vi "test_read_digital_worker.vi"() -> ()   [LabVIEW 2017]
uses:
  hardware/hardware_type.ctl
  support/Message Queue/Enqueue Message (Single).vi
  <vilib>/Utility/error.llb/Error Cluster From Error Code.vi
  <vilib>/ErrorRing/Error Ring.xnode
  measurement_data/MeasurementDatalvclass.lvclass
  support/Message Queue/Message Queue.lvlib
  support/User Event - Stop/User Event - Stop.lvlib
  logger/logger.lvlib
  hardware/Hardware.lvclass
panel:
  in  "hardware type":T1
  out "time_stamp":timestamp
  out "raw_data":u16[][](array[numeric])
  in  "stop":bool
  in  "Play Button":bool
  out "status":string
  in  "Exit":bool
  # "row is channel and col is sample / channel"
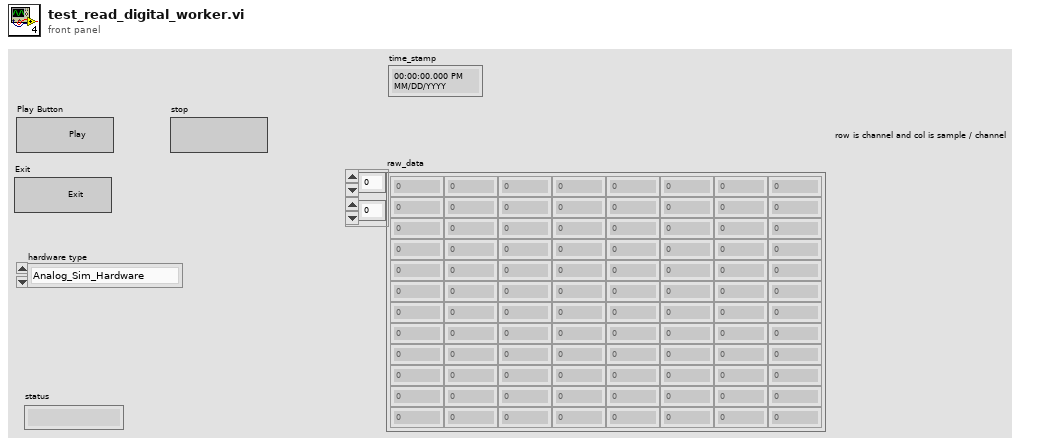
[diagram p1: front panel]
types:
  T1 = typedef "Hardware.lvclass/hardware_type.ctl" = enum16{"Analog_Sim_Hardware", "Digital_Sim_Hardware", "AI_Ni_Hardware", "AO_Ni_Hardware", "DI_Ni_Hardware", "DO_Ni_Hardware"}
  T2 = typedef "Message Queue.lvlib/All Message Queues.ctl" = cluster{"MHL":refnum<queue>, "TCPServerLoop":refnum<queue>, "RequestProcessorLoop":refnum<queue>, "AnalogReadWorkerLoop":refnum<queue>, "AnalogWriteWorkerLoop":refnum<queue>, "DigitalReadWorkerLoop":refnum<queue>, "DigitalWriteWorkerLoop":refnum<queue>}
  T3 = typedef "Notifiers.ctl" = cluster{"TCPServerExit":refnum<notifier>, "RequestProcesscorExit":refnum<notifier>, "AnalogReadWorkerrExit":refnum<notifier>, "AnalogWriteWorkerrExit":refnum<notifier>, "DigitalReadWorkerrExit":refnum<notifier>, "DigitalWriteWorkerrExit":refnum<notifier>}
  T4 = typedef "data_Notifiers.ctl" = cluster{"AnalogReadResult":refnum<notifier>}
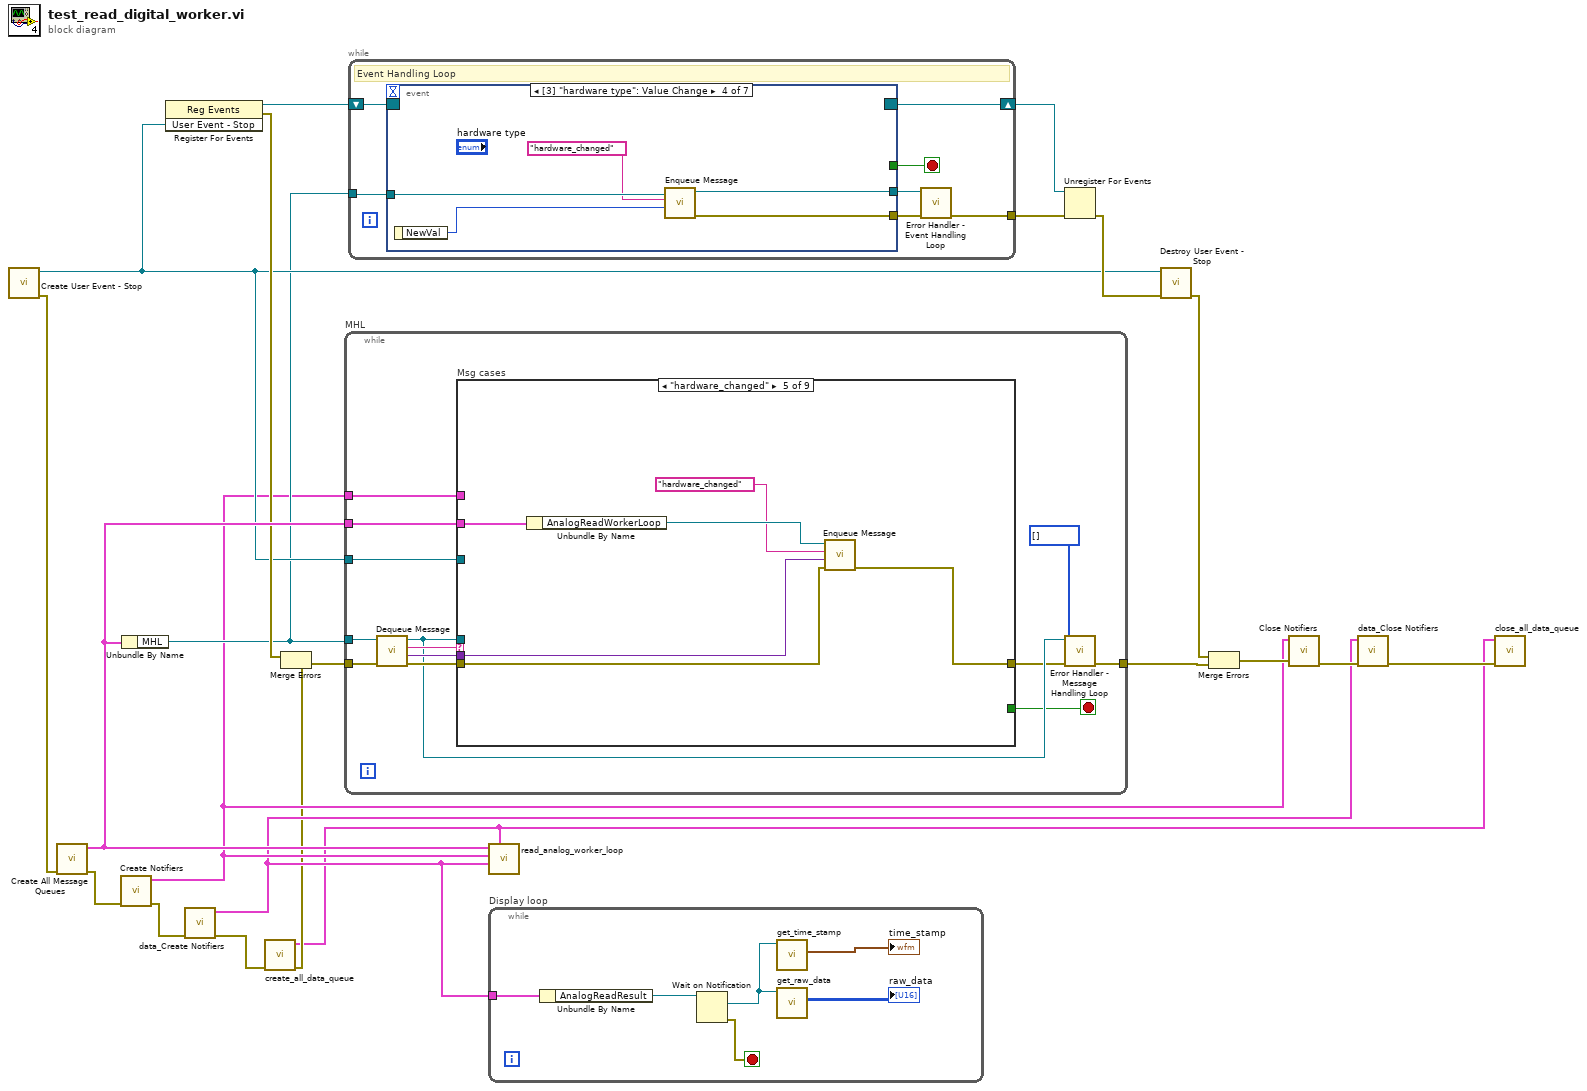
[diagram p0: block diagram]
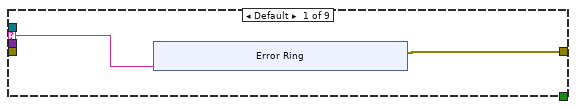
[diagram p2: hidden frame]
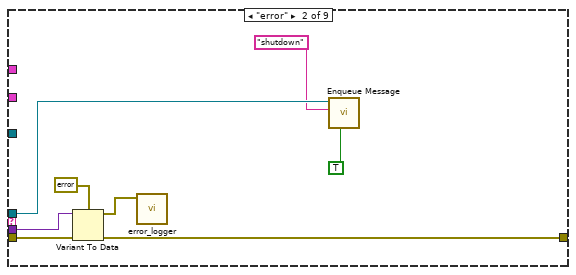
[diagram p3: hidden frame]
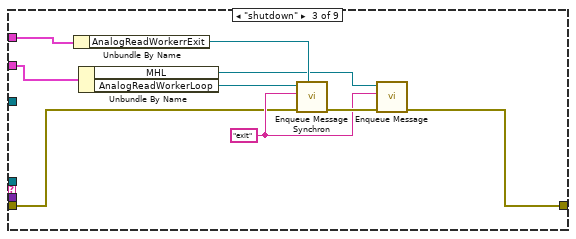
[diagram p4: hidden frame]
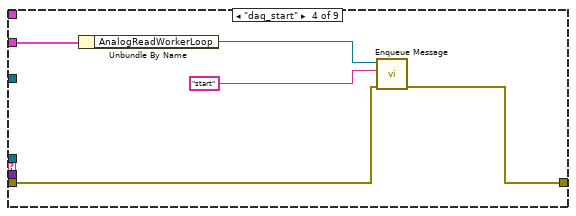
[diagram p5: hidden frame]
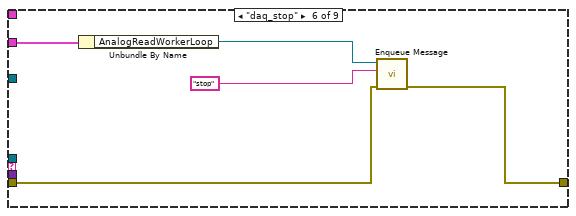
[diagram p6: hidden frame]
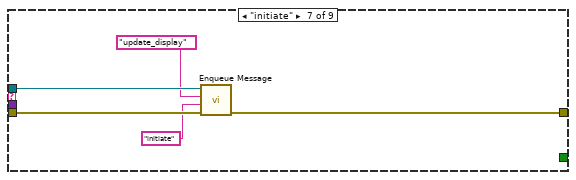
[diagram p7: hidden frame]
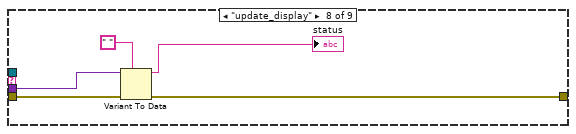
[diagram p8: hidden frame]
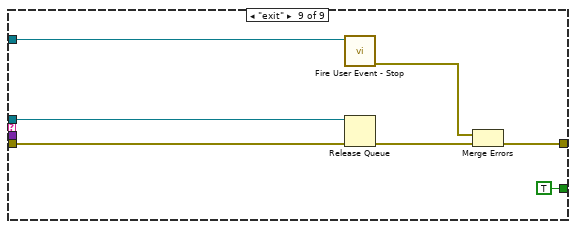
[diagram p9: hidden frame]
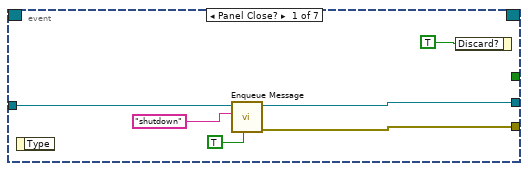
[diagram p10: hidden frame]
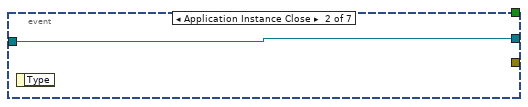
[diagram p11: hidden frame]
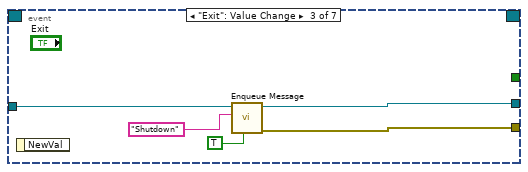
[diagram p12: hidden frame]
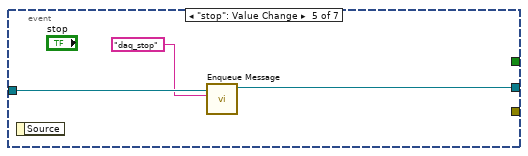
[diagram p13: hidden frame]
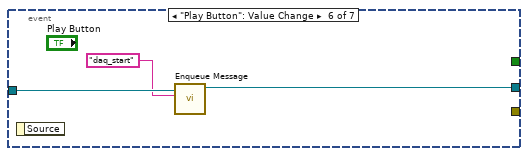
[diagram p14: hidden frame]
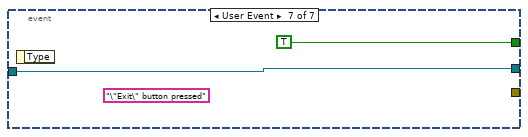
[diagram p15: hidden frame]
diagram:
  n1 = call "Create User Event - Stop.vi"() -> ("error out"=w17:errorcluster, "User Event - Stop"=w12:refnum<user-event>)  [unwired: 10 in]
  n2 = call "Create All Message Queues.vi"("error in (no error)"=w17) -> ("error out"=w16:errorcluster, "Message Queues out"=w18:T2)  [unwired: 9 in]
  n3 = call "Create Notifiers.vi"("error in"=w16) -> ("error out"=w15:errorcluster, "Notifiers"=w6:T3)  [unwired: 9 in]
  n4 = Unbundle By Name(w18) -> ("MHL"=w11:refnum<queue>)
  n5 = register-events(w12) -> (reference out=w21:refnum<event-registration>, error out=w13:errorcluster)  [unwired: 2 in]
  n6 = call "data_Create Notifiers.vi"("error in"=w15) -> ("error out"=w4:errorcluster, "output cluster"=w5:T4)  [unwired: 9 in]
  n7 = call "create_all_data_queue.vi"("error in (no error)"=w4) -> ("error out"=w3:errorcluster, "data_queue"=w1:cluster{"AnalogReadData":refnum<queue>})  [unwired: 9 in]
  n8 = Merge Errors(w13, w3) -> (w14:errorcluster)
  n9 = while "MHL" {
    tunnel: w14 -> [w32]
    tunnel: w11 -> [w31]
    tunnel: w18 -> [w30]
    tunnel: w12 -> [w29]
    tunnel: w6 -> [w25]
    tunnel: [w24] -> w8
    stop <- w26 stop-if-true
    n10 = call "Dequeue Message.vi"("error in (no error)"=w32, "Message Queue"=w31) -> ("error out"=w33:errorcluster, "Message Data"=w34:variant, "Message"=w35:string, "dup Message Queue"=w28:refnum<queue>)  [unwired: 6 in]
    n11 = case "Msg cases" shown="\"hardware_changed\"" w35 {
      selector: w35 -> [w37 _ _ _ _ _ _ _ _]
      tunnel: w28 -> [_ w52 _ _ _ _ w79 _ w92]
      tunnel: w34 -> [_ w47 _ _ w67 _ _ w85 _]
      tunnel: w33 -> [_ w46 w53 w62 w68 w73 w82 w87 w93]
      tunnel: w30 -> [_ _ w59 w66 w72 w77 _ _ _]
      tunnel: w29 -> [_ _ _ _ _ _ _ _ w91]
      tunnel: [w36 w45 w54 w63 w69 w74 w81 w86 w88] -> w27
      tunnel: [_ _ _ _ _ _ _ _ TRUE] -> w26
      tunnel: w25 -> [_ _ w61 _ _ _ _ _ _]
      frame Default {
        n12 = xnode "Error Ring"("parameter 0"=w37) -> ("error out"=w36:errorcluster)
      }
      frame "error" {
        n13 = Variant To Data(error in=w46, type=errorcluster {"status"=FALSE, "code"=0, "source"=""} ("error constant"), Variant=w47) -> (data=w48:errorcluster, error out=w45:errorcluster)
        n14 = call "error_logger.vi"("error in (no error)"=w48) -> ()  [unwired: 11 in]
        n15 = call-poly "Enqueue Message.vi"("Priority Message? (F)"=TRUE, "Message"="shutdown", "Message Queue"=w52) -> ()  [unwired: 7 in, 2 out]
      }
      frame "shutdown" {
        w55 = "exit"
        n16 = Unbundle By Name(w61) -> ("AnalogReadWorkerrExit"=w60:refnum<notifier>)
        n17 = Unbundle By Name(w59) -> ("MHL"=w57:refnum<queue>, "AnalogReadWorkerLoop"=w58:refnum<queue>)
        n18 = call "Enqueue Message Synchron.vi"("Notifier"=w60, "error in (no error)"=w53, "Message"=w55, "Message Queue"=w58) -> ("error out"=w56:errorcluster)  [unwired: 6 in, 1 out]
        n19 = call-poly "Enqueue Message.vi"("error in (no error)"=w56, "Message"=w55, "Message Queue"=w57) -> ("error out"=w54:errorcluster)  [unwired: 7 in, 1 out]
      }
      frame "daq_start" {
        n20 = Unbundle By Name(w66) -> ("AnalogReadWorkerLoop"=w65:refnum<queue>)
        n21 = call-poly "Enqueue Message.vi"("error in (no error)"=w62, "Message"="start", "Message Queue"=w65) -> ("error out"=w63:errorcluster)  [unwired: 7 in, 1 out]
      }
      frame "hardware_changed" {
        n22 = Unbundle By Name(w72) -> ("AnalogReadWorkerLoop"=w71:refnum<queue>)
        n23 = call-poly "Enqueue Message.vi"("error in (no error)"=w68, "Message Data"=w67, "Message"="hardware_changed", "Message Queue"=w71) -> ("error out"=w69:errorcluster)  [unwired: 6 in, 1 out]
      }
      frame "daq_stop" {
        n24 = Unbundle By Name(w77) -> ("AnalogReadWorkerLoop"=w76:refnum<queue>)
        n25 = call-poly "Enqueue Message.vi"("error in (no error)"=w73, "Message"="stop", "Message Queue"=w76) -> ("error out"=w74:errorcluster)  [unwired: 7 in, 1 out]
      }
      frame "initiate" {
        n26 = call-poly "Enqueue Message.vi"("error in (no error)"=w82, "Message Data"="initiate" ("status"), "Message"="update_display", "Message Queue"=w79) -> ("error out"=w81:errorcluster)  [unwired: 6 in, 1 out]
      }
      frame "update_display" {
        n27 = Variant To Data(error in=w87, type=" ", Variant=w85) -> (data=→"status":string, error out=w86:errorcluster)
      }
      frame "exit" {
        n28 = call "Fire User Event - Stop.vi"("User Event - Stop"=w91) -> ("error out"=w90:errorcluster)  [unwired: 10 in]
        n29 = Release Queue(queue=w92, error in (no error)=w93) -> (error out=w89:errorcluster)  [unwired: 1 in, 2 out]
        n30 = Merge Errors(w90, w89) -> (w88:errorcluster)
      }
    }
    n31 = call "Error Handler - Message Handling Loop.vi"("error in (no error)"=w27, "Ignore Errors (Runtime)"=i32[] [], "Message Queue"=w28) -> ("dup error in"=w24:errorcluster)  [unwired: 7 in, 1 out]
  }
  n32 = while {
    shift-right: [w96] -> w19
    shift-left: w21 -> [w97]
    tunnel: [w98] -> w22
    tunnel: w11 -> [w95]
    stop <- w100 stop-if-true
    # "Event Handling Loop"
    n33 = event shown="[3] \"hardware type\": Value Change" {
      selector: w97 -> [_ _ _ _ _ _ _]
      dyn-events: [_ _ _ _ _ _ _] -> w96
      timeout: _ -> [_ _ _ _ _ _ _]
      tunnel: [_ _ _ _ _ _ TRUE ("Discard?")] -> w100
      tunnel: [w106 _ w113 w114 _ _ _] -> w101
      tunnel: [w105 w108 w112 w115 w120 w122 w125] -> w99
      tunnel: w95 -> [w102 w108 w109 w118 w121 w124 w125]
      event Panel Close? {
        n34 = event-data() -> ()  [unwired: 1 in, 1 out]
        n35 = call-poly "Enqueue Message.vi"("Priority Message? (F)"=TRUE, "Message"="shutdown", "Message Queue"=w102) -> ("error out"=w106:errorcluster, "dup Message Queue"=w105:refnum<queue>)  [unwired: 7 in]
        n36 = event-data("Discard?"=TRUE) -> ()  [unwired: 1 in, 1 out]
      }
      event Application Instance Close {
        n37 = event-data() -> ()  [unwired: 1 in, 1 out]
      }
      event "Exit": Value Change {
        n38 = event-data() -> ()  [unwired: 1 in, 1 out]
        n39 = call-poly "Enqueue Message.vi"("Priority Message? (F)"=TRUE, "Message"="Shutdown", "Message Queue"=w109) -> ("error out"=w113:errorcluster, "dup Message Queue"=w112:refnum<queue>)  [unwired: 7 in]
      }
      event Value Change {
        n40 = event-data() -> ("NewVal"=w116:T1)  [unwired: 1 in]
        n41 = call-poly "Enqueue Message.vi"("Message Data"=w116, "Message"="hardware_changed", "Message Queue"=w118) -> ("error out"=w114:errorcluster, "dup Message Queue"=w115:refnum<queue>)  [unwired: 7 in]
      }
      event "stop": Value Change {
        n42 = event-data() -> ()  [unwired: 1 in, 1 out]
        n43 = call-poly "Enqueue Message.vi"("Message"="daq_stop", "Message Queue"=w121) -> ("dup Message Queue"=w120:refnum<queue>)  [unwired: 8 in, 1 out]
      }
      event "Play Button": Value Change {
        n44 = event-data() -> ()  [unwired: 1 in, 1 out]
        n45 = call-poly "Enqueue Message.vi"("Message"="daq_start", "Message Queue"=w124) -> ("dup Message Queue"=w122:refnum<queue>)  [unwired: 8 in, 1 out]
      }
      event User Event {
        (unwired) "\"Exit\" button pressed" ("VI Stopped")
        n46 = event-data() -> ()  [unwired: 1 in, 1 out]
      }
    }
    n47 = call "Error Handler - Event Handling Loop.vi"("error in (no error)"=w101, "Message Queue"=w99) -> ("dup error in"=w98:errorcluster)  [unwired: 8 in, 1 out]
  }
  n48 = call "read_analog_worker_loop.vi"("data_queues"=w1, "data_notifiers"=w5, "Notifiers"=w6, "Message Queues"=w18) -> ()  [unwired: 7 in, 1 out]
  n49 = while "Display loop" {
    tunnel: w5 -> [w132]
    stop <- w130 stop-if-true
    n50 = Unbundle By Name(w132) -> ("AnalogReadResult"=w131:refnum<notifier>)
    n51 = Wait on Notification(notifier=w131) -> (notification=w128:refnum<class "MeasurementDatalvclass.lvclass">, error out=w130:errorcluster)  [unwired: 3 in, 2 out]
    n52 = call "get_time_stamp.vi"("MeasurementResult in"=w128) -> ("time_stamp"=→"time_stamp":timestamp)  [unwired: 8 in, 2 out]
    n53 = call-dynamic "get_raw_data.vi"("MeasurementResult in"=w128) -> ("raw_data"=→"raw_data":u16[][])  [unwired: 8 in, 2 out]
  }
  n54 = Unregister For Events(event registration refnum=w19, error in=w22) -> (error out=w20:errorcluster)
  n55 = call "Destroy User Event - Stop.vi"("error in (no error)"=w20, "User Event - Stop"=w12) -> ("error out"=w9:errorcluster)  [unwired: 9 in]
  n56 = Merge Errors(w9, w8) -> (w7:errorcluster)
  n57 = call "Close Notifiers.vi"("error in"=w7, "Notifiers"=w6) -> ("error out"=w10:errorcluster)  [unwired: 9 in]
  n58 = call "data_Close Notifiers.vi"("error in"=w10, "Data Notifiers"=w5) -> ("error out"=w2:errorcluster)  [unwired: 9 in]
  n59 = call "close_all_data_queue.vi"("error in (no error)"=w2, "data_queue"=w1) -> ()  [unwired: 9 in, 1 out]
